vi "DWF MSO Initialize.vi"(0 "Device Name":string, 5 "Reset":bool=TRUE caption="Reset (True)", 11 "Error In":errorcluster caption="Error In (no error)") -> (4 "Instrument Handle Out":u32, 15 "Error Out":errorcluster)   [LabVIEW 2015, in "DigilentWF.lvlib"]
doc: "Establishes communication with the device. This VI should be called once per session."
uses:
  <vilib>/DigilentWF/DigilentWF.lvlib
  dwf.dll
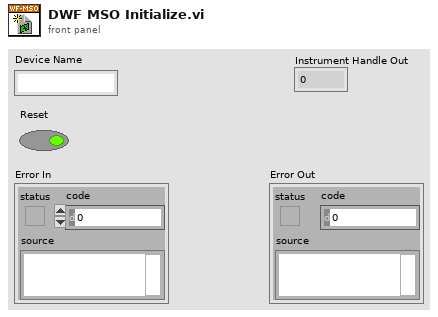
[diagram p1: front panel]
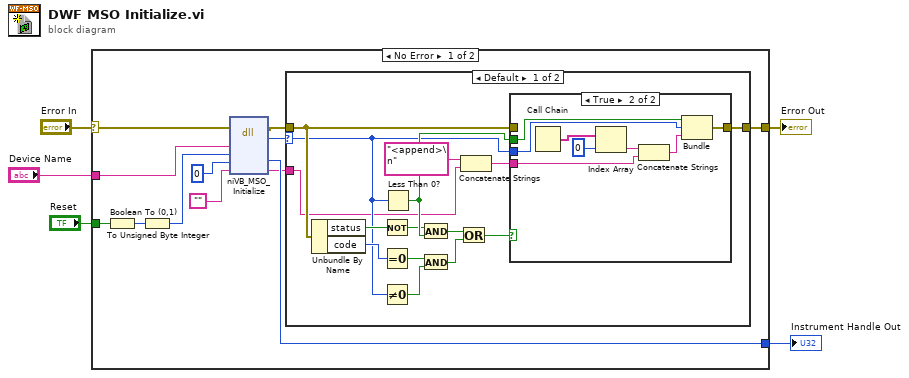
[diagram p0: block diagram]
diagram:
  n1 = case "outter_case" shown="No Error" "Error In" {
    selector: "Error In" -> [w14 w43]
    tunnel: [w17 w43] -> w4
    tunnel: "Device Name" -> [w12 _]
    tunnel: "Reset" -> [w15 _]
    tunnel: [w10 _] -> w1
    frame No Error {
      n2 = Boolean To (0,1)(Boolean=w15) -> (0, 1=w16:i16)
      n3 = To Unsigned Byte Integer(number=w16) -> (unsigned 8bit integer=w11:u8)
      n4 = dll-call lib="dwf.*" fn="niVB_MSO_Initialize"(error in=w14, "deviceName"=w12, "reset"=w11, "instrumentHandle"=u32 0, "szError"="") -> (error out=w13:errorcluster, "return type"=w9:i32, "instrumentHandle"=w10:u32, "szError"=w7:string)  [unwired: 4 in, 1 out]
      n5 = case "inner_case" shown="Default" w9 {
        selector: w9 -> [w22 _]
        tunnel: w13 -> [w23 w42]
        tunnel: [w19 w42] -> w17
        tunnel: w7 -> [w18 _]
        frame Default {
          n6 = Unbundle By Name(w23) -> ("status"=w27:bool, "code"=w31:i32)
          n7 = Not(x=w27) -> (.not. x?=w30:bool)
          n8 = Equal To 0?(x=w31) -> (x = 0?=w26:bool)
          n9 = Not Equal To 0?(x=w22) -> (x != 0?=w29:bool)
          n10 = Less Than 0?(x=w22) -> (x < 0?=w32:bool)
          n11 = And(x=w30, y=w32) -> (x .and. y?=w28:bool)
          n12 = And(x=w26, y=w29) -> (x .and. y?=w25:bool)
          n13 = Or(x=w28, y=w25) -> (x .or. y?=w24:bool)
          n14 = Concatenate Strings("<append>\n" ("string"), w18) -> (w21:string)
          n15 = case shown="True" w24 {
            tunnel: [w33 w40] -> w19
            tunnel: w22 -> [_ w39]
            tunnel: w32 -> [_ w38]
            tunnel: w23 -> [w33 _]
            tunnel: w21 -> [_ w34]
            frame False {
            }
            frame True {
              n16 = Call Chain() -> (call chain=w37:string[])
              n17 = Index Array(array=w37, index=0) -> (element=w36:string)
              n18 = Concatenate Strings(w36, w34) -> (w41:string)
              n19 = Bundle(w38, "return type"=w39, w41) -> (w40:cluster{bool, "return type":i32, string})  [unwired: 1 out]
            }
          }
        }
        frame 0 {
        }
      }
    }
    frame Error {
    }
  }
  "Error Out" <- w4
  "Instrument Handle Out" <- w1
